vi "Shooter Controller.vi"(8 "error in":errorcluster) -> ()   [LabVIEW 2015]
doc: "This VI executes continuously carrying out the current operation and responding to updates or new operations. It will often contain the timing or control code that is difficult to place directly in TeleOp. This VI generally opens all sensors and motors and isolates the rest of the robot code from knowing how the operations are carried out."
uses:
  Shooter Operations.ctl
  Shooter Setpoints.ctl
  <vilib>/Rock Robotics/WPI/MotorControl/WPI_MotorControlOpen.vi
  <vilib>/Rock Robotics/WPI/CAN/TalonSRX/WPI_CANTalonSRX_APIControlMode.ctl
  <vilib>/Rock Robotics/WPI/MotorControl/WPI_MotorControlOpenCANTalonSRX.vi
  <vilib>/Rock Robotics/WPI/CAN/TalonSRX/WPI_CANTalonSRX_APIFeedbackSelect.ctl
  <vilib>/addons/control/pid/NI_PID_pid.lvlib
  <vilib>/Rock Robotics/WPI/CAN/TalonSRX/WPI_CANTalonSRX_BrakeOverride.ctl
  <vilib>/addons/control/pid/pid.llb/PID (DBL).vi
  <vilib>/Rock Robotics/Network Tables/NT Write Boolean.vi
  Shooter Published Globals.vi
  Framework/Robot Global Data.vi
panel:
  in  "PID Gains":T1={"proportional gain (Kc)"=0.6, "integral time (Ti, min)"=0.0, "derivative time (Td, min)"=0.0} {"derivative time (Td, min)" format="%.3f"; "integral time (Ti, min)" format="%.3f"; "proportional gain (Kc)" format="%.3f"}
  out "SHOOTER BROKEN":bool
  in  "Distance to Motor Speed Conversions":dbl[](array[numeric])
  out "Current\nCmd":string
  # "Tip: It may be helpful to observe inputs and sensor values.\nYou may also want to display tuning or debugging controls."
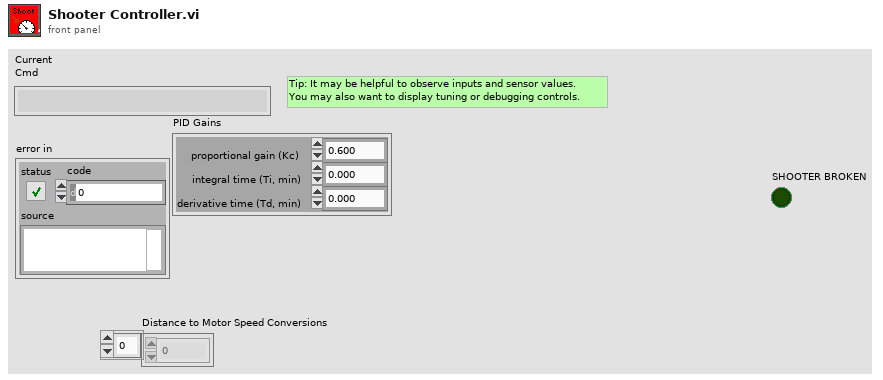
[diagram p1: front panel]
types:
  T1 = cluster{"proportional gain (Kc)":dbl, "integral time (Ti, min)":dbl, "derivative time (Td, min)":dbl}
  T2 = typedef "WPI_CANTalonSRX_BrakeOverride.ctl" = enum8{"No Override", "Override to Coast", "Override to Brake"}
  T3 = typedef "WPI_CANTalonSRX_APIControlMode.ctl" = enum8{"Percent VBus", "Speed", "Position", "Slave", "Unchanged / Invalid", "Voltage Compensation", "Current", "Motion Profile"}
  T4 = typedef "WPI_CANTalonSRX_APIFeedbackSelect.ctl" = enum16{"Digital Quadrature Encoder", "Analog Potentiometer", "Analog Encoder", "Count on Quad-A (Rising-Edge)", "Count on Quad-A (Falling-Edge)", "CTR Magnetic Enc (Absolute)", "CTR Magnetic Enc (Relative)", "Pulse Width"}
  T5 = typedef "Shooter Setpoints.ctl" = cluster{"Operation":T6, "Setpoint":dbl, "Duration":dbl}
  T6 = typedef "Shooter Operations.ctl" = enum16{"Reserve", "Read Current", "Immediate", "Fire", "Aim"}
  T7 = typedef "WPI_MotorControlDeviceRef.ctl" = cluster{"DeviceStatus":errorcluster, "Type":T8, "PWM":cluster{"PWM Channel":T9, "DeadBand":T10}, "CAN":cluster{"Device Number":u8, "Control Mode":T11, "Semaphore":T12, "Max Vout":dbl, "TalonSRX Control Mode":T3}, "Invert":bool}
  T8 = typedef "WPI_MotorControlType.ctl" = enum16{"PWM", "CAN", "CANTalonSRX"}
  T9 = typedef "FPGA_DIOPWMChannel.ctl" = enum8{"PWM 0", "PWM 1", "PWM 2", "PWM 3", "PWM 4", "PWM 5", "PWM 6", "PWM 7", "PWM 8", "PWM 9", "PWM MXP 0", "PWM MXP 1", "PWM MXP 2", "PWM MXP 3", "PWM MXP 4", "PWM MXP 5", "PWM MXP 6", "PWM MXP 7", "PWM MXP 8", "PWM MXP 9", "Invalid"}
  T10 = typedef "WPI_PWMDeadband.ctl" = cluster{"Name":string, "maxPositivePwm":i32, "minPositivePwm":i32, "centerPwm":i32, "maxNegativePwm":i32, "minNegativePwm":i32, "angularRange":u16}
  T11 = typedef "WPI_CANJaguar_ControlMode.ctl" = enum8{"Percent VBus", "Current", "Speed", "Position", "Voltage"}
  T12 = typedef "Semaphore RefNum" = refnum<k1>
  T13 = typedef "Command Status Info.ctl" = cluster{"Name":string, "Status":T14, "notifier out":T15}
  T14 = typedef "Completion Status.ctl" = enum16{"Successful", "Aborted", "Incomplete"}
  T15 = typedef "Completion Notifier.ctl" = refnum<notifier>
  T16 = cluster{"Default Command":T5, "Command Timing":cluster{"Start Time (ms)":u32, "Iterations":i32}, "Command Arguments":cluster{"Command Info":T13, "Description":string, "Default Command":T5, "notifier out":refnum<notifier>, "Subsystem Name":string}}
  T17 = typedef "WPI_CANTalonSRX_GlobalStatus.ctl" = cluster{"Applied Throttle":dbl, "Module Enabled":bool, "CAN Error":errorcluster, "Closed Loop Error":dbl, "Forward Limit Switch Closed":bool, "Reverse Limit Switch Closed":bool, "Sensor Position":dbl, "Sensor Velocity":dbl, "Current":dbl, "Sticky Fault - Over Temp":bool, "Sticky Fault - Under Voltage":bool, "Sticky Fault - Forward Limit":bool, "Sticky Fault - Reverse Limit":bool, "Sticky Fault - Forward Soft Limit":bool, "Sticky Fault - Reverse Soft Limit":bool, "Brake is Enabled":bool, "Encoder Position":dbl, "Encoder Velocity":dbl, "Encoder Index Count":dbl, "Encoder A Pin State":bool, "Encoder B Pin State":bool, "Encoder Index Pin State":bool, "Analog In":dbl, "Analog In Velocity":dbl, "Temperature (C)":dbl, "Battery Voltage":dbl, "Control 5 Is Supported":bool, "Current Profile Slot Select":dbl, "Pos Div 8":bool, "Vel Div 4":bool, "Pulse Width Position":i32, "Pulse Width Velocity":i32, "Pulse Width Rise To Rise (us)":i32, "Pulse Width Rise To Fall (us)":i32, "Mot Prof Active Is Under Run":bool, "Mot Prof Active Has Under Run":bool, "Mot Prof Active Is Last":bool, "Mot Prof Active Velocity Only":bool, "Mot Prof Active Is Valid":bool, "Mot Prof Buffer Is Full":bool, "Mot Prof Active Profile Slot Select":i32, "Mot Prof NextID":i32, "Mot Prof Count":i32, "Mot Prof Active Velocity":dbl, "Mot Prof Active Position":dbl, "Mot Prof Output Enable":i32}
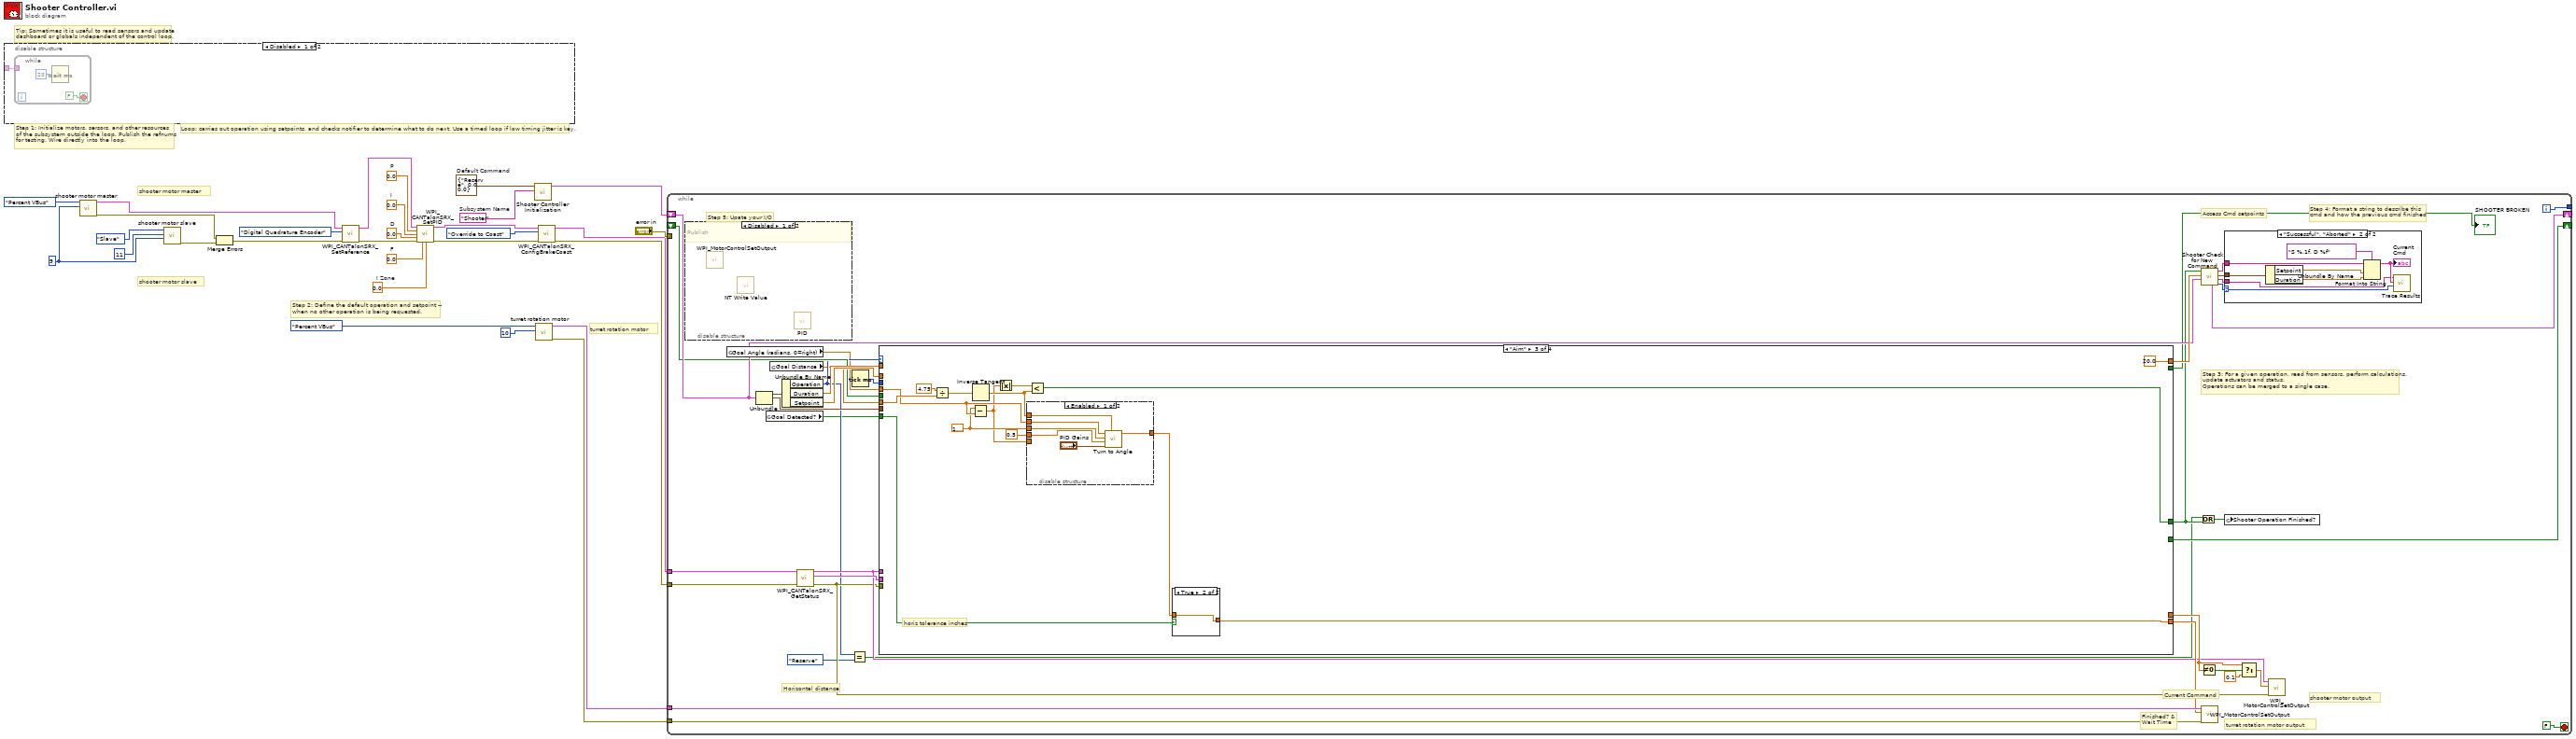
[diagram p0: block diagram]
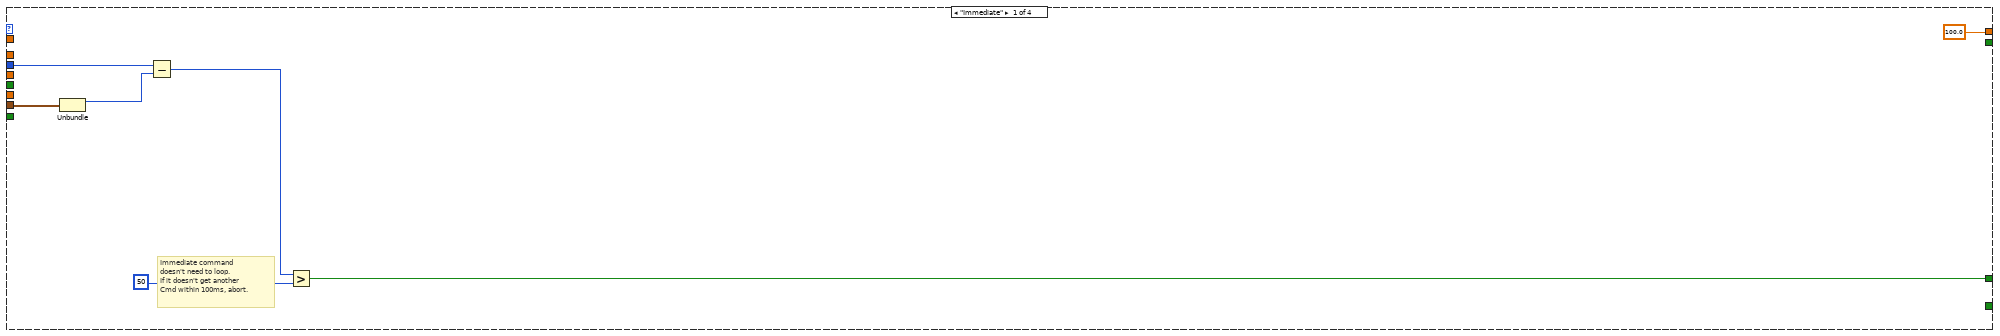
[diagram p5: hidden frame]
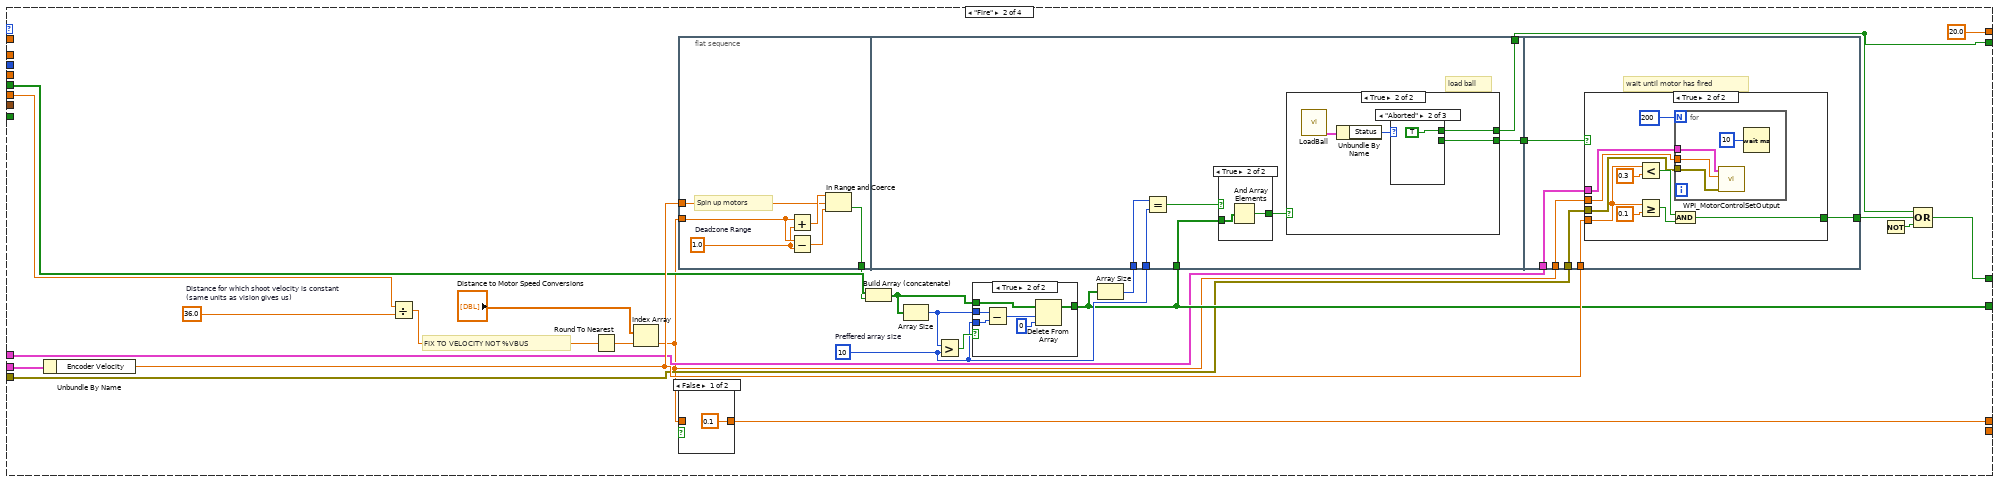
[diagram p6: hidden frame]
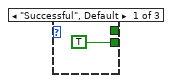
[diagram p11: hidden frame]
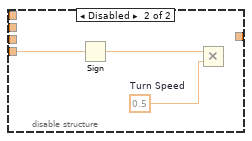
[diagram p14: hidden frame]
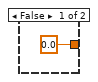
[diagram p15: hidden frame]
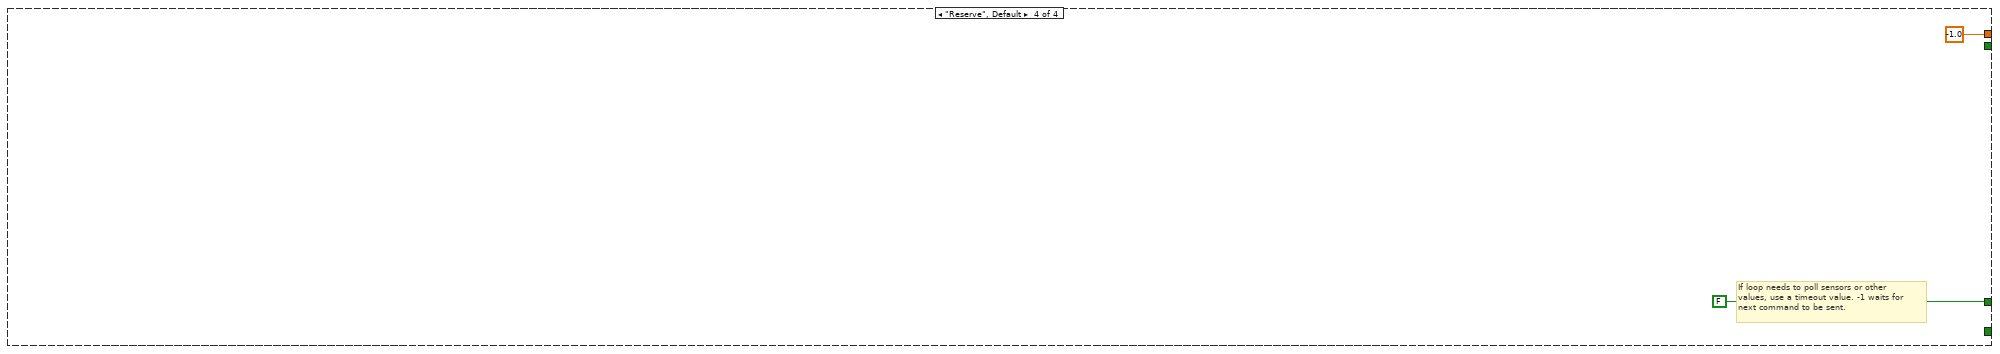
[diagram p16: hidden frame]
diagram:
  w1 = 0.0  # F
  w2 = 0.0  # I Zone
  w3 = 0.0  # D
  w4 = 0.0  # I
  w5 = 0.0  # P
  w16 = u8 9 ("Master Device Number")
  w26 = T5 {"Operation"=enum."Reserve", "Setpoint"=0.0, "Duration"=0.0}  # Default Command
  w27 = "Shooter"  # Subsystem Name
  # "turret rotation motor"
  # "shooter motor slave"
  # "shooter motor master"
  # "Tip: Sometimes it is useful to read sensors and update\ndashboard or globals independent of the control loop."
  # "Step 2: Define the default operation and setpoint --\nwhen no other operation is being requested."
  # "Step 1: Initialize motors, sersors, and other resources\nof the subsystem outside the loop. Publish the refnums\nfor testing. Wire directly into the loop."
  # "Loop: carries out operation using setpoints, and checks notifier to determine what to do next. Use a timed loop if low timing jitter is key."
  n1 = disable-structure shown="Disabled" {
    disable-tunnel: _ -> [w30 _]
    frame Disabled {
      n2 = while {
        tunnel: w30 -> [_]
        stop <- FALSE stop-if-true
        n3 = Wait (ms)(milliseconds to wait=u32 20) -> ()  [unwired: 1 out]
      }
    }
    frame Enabled {
    }
  }
  n4 = call-poly "shooter motor master"("Device Number"=w16, "Control Mode"=WPI_CANTalonSRX_APIControlMode."Percent VBus") -> ("error out"=w15:errorcluster, "MotorControlDeviceRef"=w22:T7)  [unwired: 8 in]
  n5 = call-poly "shooter motor slave"("Master Device Number"=w16, "Device Number"=u8 11 ("Master Device Number"), "Control Mode"=WPI_CANTalonSRX_APIControlMode."Slave") -> ("error out"=w14:errorcluster)  [unwired: 7 in, 1 out]
  n6 = Merge Errors(w15, w14) -> (w13:errorcluster)
  n7 = call <vilib>:"WPI_CANTalonSRX_SetReference.vi"("error in (no error)"=w13, "Feedback Reference"=WPI_CANTalonSRX_APIFeedbackSelect."Digital Quadrature Encoder", "CAN Talon SRX Ref"=w22) -> ("error out"=w11:errorcluster, "CAN Talon SRX Ref"=w8:T7)  [unwired: 7 in]
  n8 = call <vilib>:"WPI_CANTalonSRX_SetPID.vi"("CAN Talon SRX Ref"=w8, "P"=w5, "I"=w4, "D"=w3, "error in (no error)"=w11, "F"=w1, "I Zone"=w2) -> ("CAN Talon SRX Ref"=w7:T7, "error out"=w10:errorcluster)  [unwired: 7 in]
  n9 = call "Shooter Controller Initialization.vi"("Subsystem Name"=w27, "Default Command"=w26) -> ("Command Info"=w28:T16)  [unwired: 9 in]
  n10 = call-poly "turret rotation motor"("Device Number"=u8 10 ("Master Device Number"), "Control Mode"=WPI_CANTalonSRX_APIControlMode."Percent VBus") -> ("error out"=w19:errorcluster, "MotorControlDeviceRef"=w24:T7)  [unwired: 8 in]
  n11 = call <vilib>:"WPI_CANTalonSRX_ConfigBrakeCoast.vi"("error in (no error)"=w10, "Brake / Coast Mode"=WPI_CANTalonSRX_BrakeOverride."Override to Coast", "CAN Talon SRX Ref"=w7) -> ("error out"=w9:errorcluster, "CAN Talon SRX Ref"=w12:T7)  [unwired: 7 in]
  n12 = while {
    shift-right: [w62] -> _
    shift-left: w28 -> [w53]
    tunnel: [w68] -> _
    tunnel: "error in" -> [_]
    tunnel: w24 -> [w56]
    tunnel: w12 -> [w52]
    tunnel: w19 -> [w55]
    tunnel: w9 -> [w51]
    shift-right: [w45] -> _
    shift-left: _ -> [w46]
    i -> [w68]
    stop <- FALSE stop-if-true
    # "Horizontal distance"
    # "shooter motor output"
    # "turret rotation motor output"
    # "Step 5: Upate your I/O"
    # "Step 4: Format a string to describe this\ncmd and how the previous cmd finished"
    # "Current Command"
    # "Access Cmd setpoints"
    # "Finished? &\nWait Time"
    # "Step 3: For a given operation, read from sensors, perform calculations,\nupdate actuators and status.\nOperations can be merged to a single case."
    n13 = disable-structure shown="Disabled" {
      frame Disabled {
        # "Publish"
        n14 = call <vilib>:"WPI_MotorControlSetOutput.vi"() -> ()  [unwired: 9 in, 3 out]
        n15 = call-poly <vilib>:"NT Write Value.vi"() -> ()  [unwired: 11 in, 1 out]
        n16 = call-poly <vilib>:"PID.vi"() -> ()  [unwired: 10 in, 2 out]
      }
      frame Enabled {
      }
    }
    n17 = global read "Robot Global Data.vi" "Goal Angle (radians, 0=right)"() -> (w33:dbl)
    n18 = Unbundle(w53) -> ("Default Command"=w67:T5, "Command Timing"=w64:cluster{"Start Time (ms)":u32, "Iterations":i32})  [unwired: 1 out]
    n19 = global read "Robot Global Data.vi" "Goal Detected?"() -> (w35:bool)
    n20 = global read "Robot Global Data.vi" "Goal Distance"() -> (w34:dbl)
    n21 = Unbundle By Name(w67) -> ("Operation"=w38:T6, "Duration"=w66:dbl, "Setpoint"=w63:dbl)
    n22 = call <vilib>:"WPI_CANTalonSRX_GetStatus.vi"("error in (no error)"=w51, "CAN Talon SRX Ref"=w52) -> ("error out"=w41:errorcluster, "Talon SRX Status"=w50:T17, "CAN Talon SRX Ref"=w42:T7)  [unwired: 7 in]
    n23 = Equal?(x=w38, y=Shooter_Operations."Reserve") -> (x = y?=w39:bool)
    n24 = Tick Count (ms)() -> (millisecond timer value=w65:u32)
    n25 = case shown="\"Aim\"" w38 {
      tunnel: [100.0 20.0 20.0 -1.0] -> w61
      tunnel: [w78 w85 w172 FALSE ("ignore previous (F)")] -> w40
      tunnel: w64 -> [w80 _ _ _]
      tunnel: w66 -> [_ _ _ _]
      tunnel: w65 -> [w79 _ _ _]
      tunnel: w63 -> [_ _ _ _]
      tunnel: w33 -> [_ _ w165 _]
      tunnel: [_ _ w170 _] -> w54
      tunnel: w34 -> [_ w105 w167 _]
      tunnel: [_ w90 _ _] -> w43
      tunnel: w50 -> [_ w103 _ _]
      tunnel: [_ w88 _ _] -> w47
      tunnel: w46 -> [_ w100 _ _]
      tunnel: [_ w94 _ _] -> w45
      tunnel: w42 -> [_ w92 _ _]
      tunnel: w41 -> [_ w91 _ _]
      tunnel: w35 -> [_ _ w169 _]
      frame "Immediate" {
        # "Immediate command\ndoesn't need to loop.\nIf it doesn't get another\nCmd within 100ms, abort."
        n26 = Unbundle(w80) -> ("Start Time (ms)"=w83:u32)  [unwired: 1 out]
        n27 = Subtract(x=w79, y=w83) -> (x-y=w82:u32)
        n28 = Greater?(x=w82, y=u8 50 ("Left Motor")) -> (0:w78:bool)
      }
      frame "Fire" {
        w95 = 10  # Preffered array size
        w104 = 36.0  # Distance for which shoot velocity is constant  (same units as vision gives us)
        # "FIX TO VELOCITY NOT %VBUS"
        n29 = Unbundle By Name(w103) -> ("Encoder Velocity"=w102:dbl)
        n30 = Divide(x=w105, y=w104) -> (x/y=w106:dbl)
        n31 = Round To Nearest(number=w106) -> (nearest integer value=w107:dbl)
        n32 = Index Array(array="Distance to Motor Speed Conversions", index=w107) -> (element=w89:dbl)
        n33 = flat-sequence {
          tunnel: w89 -> [w122]
          tunnel: w102 -> [w121]
          tunnel: [w119] -> w99
          tunnel: [w130] -> w101
          tunnel: [w131] -> w88
          tunnel: w94 -> [w127]
          tunnel: w95 -> [w128]
          tunnel: w93 -> [w125]
          tunnel: w101 -> [w143]
          tunnel: w102 -> [w145]
          tunnel: [w144] -> w87
          tunnel: w92 -> [w142]
          tunnel: w89 -> [w141]
          tunnel: w91 -> [w140]
          frame #0 {
            w120 = 1.0  # Deadzone Range
            # "Spin up motors"
            n34 = Add(x=w122, y=w120) -> (x+y=w123:dbl)
            n35 = Subtract(x=w122, y=w120) -> (x-y=w124:dbl)
            n36 = In Range and Coerce(upper limit=w123, x=w121, lower limit=w124) -> (In Range?=w119:bool)  [unwired: 1 out]
          }
          frame #1 {
            # "load ball"
            n37 = Equal?(x=w125, y=w128) -> (x = y?=w126:bool)
            n38 = case shown="True" w126 {
              tunnel: [_ w133] -> w129
              tunnel: w127 -> [_ w132]
              frame False {
              }
              frame True {
                n39 = And Array Elements(Boolean array=w132) -> (logical AND=w133:bool)
              }
            }
            n40 = case shown="True" w129 {
              tunnel: [_ w135] -> w131
              tunnel: [_ w134] -> w130
              frame False {
              }
              frame True {
                n41 = call "LoadBall.vi"() -> ("Command Info Out"=w137:T13)  [unwired: 11 in]
                n42 = Unbundle By Name(w137) -> ("Status"=w136:T14)
                n43 = case shown="\"Aborted\"" w136 {
                  tunnel: [TRUE ("ignore previous (F)") _ _] -> w134
                  tunnel: [_ TRUE _] -> w135
                  frame "Successful", Default {
                  }
                  frame "Aborted" {
                  }
                  frame "Incomplete" {
                  }
                }
              }
            }
          }
          frame #2 {
            # "wait until motor has fired"
            n44 = case shown="True" w143 {
              tunnel: w145 -> [_ w151]
              tunnel: [_ w154] -> w144
              tunnel: w142 -> [_ w148]
              tunnel: w141 -> [_ w147]
              tunnel: w140 -> [_ w146]
              frame False {
              }
              frame True {
                n45 = Less?(x=w151, y=0.3) -> (x < y?=w152:bool)
                n46 = Greater Or Equal?(x=w151, y=0.1) -> (x >= y?=w155:bool)
                n47 = And(x=w152, y=w155) -> (x .and. y?=w154:bool)
                n48 = for {
                  N: 200 -> [_]
                  tunnel: w148 -> [w158]
                  tunnel: w147 -> [w157]
                  tunnel: w146 -> [w156]
                  n49 = call <vilib>:"WPI_MotorControlSetOutput.vi"("error in (no error)"=w156, "Output"=w157, "MotorControlDevRef"=w158) -> ()  [unwired: 6 in, 3 out]
                  n50 = Wait (ms)(milliseconds to wait=u32 10) -> ()  [unwired: 1 out]
                }
              }
            }
          }
        }
        n51 = case shown="False" {
          selector: _ -> [_ _]
          tunnel: [0.1 w111] -> w90
          tunnel: w89 -> [_ w111]
          frame False {
          }
          frame True {
          }
        }
        n52 = Build Array (concatenate)(w100, w99) -> (w97:bool[])
        n53 = Array Size(array=w97) -> (size(s)=w96:i32)
        n54 = Greater?(x=w96, y=w95) -> (0:w98:bool)
        n55 = case shown="True" w98 {
          tunnel: w97 -> [w112 w118]
          tunnel: w95 -> [_ w117]
          tunnel: w96 -> [_ w116]
          tunnel: [w112 w115] -> w94
          frame False {
          }
          frame True {
            n56 = Subtract(x=w116, y=w117) -> (x-y=w114:i32)
            n57 = Delete From Array(array=w118, length=w114, index=0) -> (array with subset deleted=w115:bool[])  [unwired: 1 out]
          }
        }
        n58 = Array Size(array=w94) -> (size(s)=w93:i32)
        n59 = Not() -> (.not. x?=w86:bool)  [unwired: 1 in]
        n60 = Compound Arithmetic op=OR(w88, w87, w86) -> (w85:bool)
      }
      frame "Aim" {
        w164 = 1.5707963267948966
        # "horiz tolerance inches"
        n61 = Divide(x=4.75 ("y"), y=w167) -> (x/y=w171:dbl)
        n62 = Subtract(x=w164, y=w165) -> (x-y=w160:dbl)
        n63 = Inverse Tangent(1:w171) -> (0:w162:dbl)
        n64 = Absolute Value(x=w160) -> (abs(x)=w166:dbl)
        n65 = disable-structure shown="Enabled" {
          disable-tunnel: w165 -> [w179 _]
          disable-tunnel: w164 -> [w178 _]
          disable-tunnel: 0.5 ("Rotation Multiplier") -> [w177 _]
          disable-tunnel: w162 -> [w175 _]
          disable-tunnel: [w174 _] -> w161
          disable-tunnel: w160 -> [_ w182]
          frame Enabled {
            n66 = call "Turn to Angle.vi"("Angle Tolerance"=w175, "PID Gains"="PID Gains", "Rotation Multiplier"=w177, "Target angle"=w178, "Angle (radians; 0 = right)"=w179) -> ("Turn Set Point"=w174:dbl)  [unwired: 2 in, 1 out]
          }
          frame Disabled {
            w180 = 0.5  # Turn Speed
            n67 = Sign(1:w182) -> (0:w181:dbl)
            n68 = Multiply(x=w181, y=w180) -> ()  [unwired: 1 out]
          }
        }
        n69 = Less?(x=w166, y=w162) -> (x < y?=w172:bool)
        n70 = case shown="True" w169 {
          tunnel: [0.0 w184] -> w170
          tunnel: w161 -> [_ w184]
          frame False {
          }
          frame True {
          }
        }
      }
      frame "Reserve", Default {
        # "If loop needs to poll sensors or other\nvalues, use a timeout value. -1 waits for\nnext command to be sent."
      }
    }
    "SHOOTER BROKEN" <- w47
    n71 = Or(x=w39, y=w40) -> (x .or. y?=w36:bool)
    n72 = Not Equal To 0?(x=w43) -> (x != 0?=w44:bool)
    n73 = call "Shooter Check for New Command.vi"("Current Command"=w53, "Wait time (ms)"=w61, "Finished?"=w40) -> ("Completion"=w57:T14, "Subsystem Name"=w58:string, "Current Command"=w59:T5, "Initial Trace String"=w60:string, "NextCommand"=w62:T16)  [unwired: 4 in]
    n74 = call <vilib>:"WPI_MotorControlSetOutput.vi"("error in (no error)"=w55, "Output"=w54, "MotorControlDevRef"=w56) -> ()  [unwired: 6 in, 3 out]
    n75 = case shown="\"Successful\", \"Aborted\"" w57 {
      selector: w57 -> [_ w77]
      tunnel: w60 -> [_ w73]
      tunnel: w59 -> [_ w74]
      tunnel: w58 -> [_ w70]
      frame "Incomplete", Default {
        # "Continuing current command"
      }
      frame "Successful", "Aborted" {
        # "Report and setup for next command"
        n76 = Unbundle By Name(w74) -> ("Setpoint"=w76:dbl, "Duration"=w71:dbl)
        n77 = Format Into String(format string="S %.1f, D %f", initial string=w73, w76, w71) -> (resulting string=w72:string)  [unwired: 1 in, 1 out]
        "Current\nCmd" <- w72
        n78 = call <vilib>:"Trace Results.vi"("Status of previous command"=w77, "Description"=w72, "Subsystem"=w70) -> ()  [unwired: 9 in]
      }
    }
    n79 = global write "Shooter Published Globals.vi" "Shooter Operation Finished?"(w36) -> ()
    n80 = Select(t=w43, s=w44, f=0.1) -> (s? t:f=w48:dbl)
    n81 = call <vilib>:"WPI_MotorControlSetOutput.vi"("error in (no error)"=w41, "Output"=w48, "MotorControlDevRef"=w42) -> ()  [unwired: 6 in, 3 out]
  }
